vi "zherk - Hermitian Matrix Rank-k Update (CDB).vi"(4 "beta":dbl=1.0, 6 "alpha":dbl=1.0, 7 "operation A":T1 items=["Direct", "Conjugated & Transposed", "Transposed"], 8 "matrix C type":T2=3 items=["Lower Triangular"=2, "Upper Triangular"=3], 9 "C":T3, 11 "A":T3) -> (0 "error":i32, 3 "zherk":T3)   [LabVIEW 2017, in "NI_AALBLAS.lvlib"]
doc: "Calculates the rank-k update of the upper or lower triangular component of a Hermitian matrix."
uses:
  <vilib>/Analysis/NI_AALBLAS.lvlib
  <vilib>/Analysis/Matrix/Datatypes/ComplexMatrix.ctl
  <vilib>/Analysis/BLAS.llb/LV_UpLo.ctl
  <vilib>/Analysis/BLAS.llb/LV_Transpose.ctl
  <vilib>/Analysis/BLAS.llb/Fucntion.ctl
  <vilib>/Analysis/BLAS.llb/Order.ctl
  <vilib>/Analysis/BLAS.llb/BLAS3 Utility(CDB).vi
  <vilib>/Analysis/Matrix/NI_Matrix.lvlib
panel:
  # "zherk=alpha*A*conjg(A')+beta*C / zherk=alpha*conjg(A')*A+beta*C"
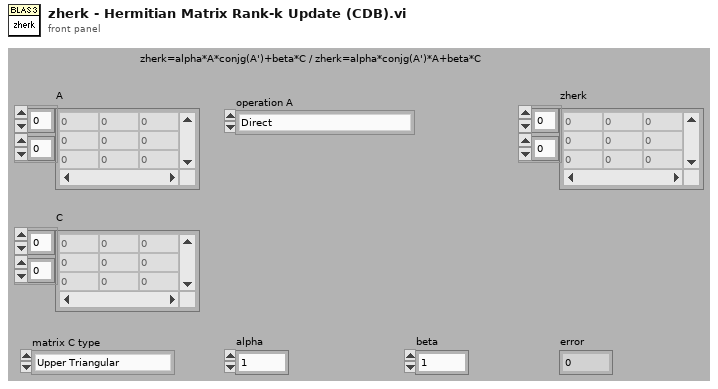
[diagram p1: front panel]
types:
  T1 = typedef "NI_AALBLAS.lvlib/LV_Transpose.ctl" = i32
  T2 = typedef "NI_AALBLAS.lvlib/LV_UpLo.ctl" = i32
  T3 = typedef "NI_Matrix.lvlib/ComplexMatrix.ctl" = cdb[][]
  T4 = typedef "NI_AALBLAS.lvlib/Order.ctl" = i32
  T5 = typedef "NI_AALBLAS.lvlib/Fucntion.ctl" = u16
  T6 = typedef "NI_AALBLAS.lvlib/Operation_Transpose.ctl" = i32
  T7 = typedef "NI_AALBLAS.lvlib/UpLo.ctl" = i32
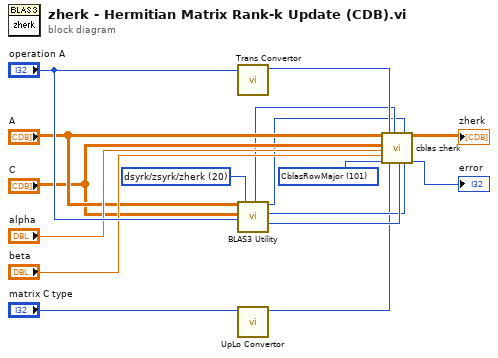
[diagram p0: block diagram]
diagram:
  w4 = T4 101 items=["CblasRowMajor"=101, "CblasColMajor"=102] ("order")
  w7 = T5 20 items=["ddot/zdotu/zdotc", "daxpy/zaxpy", "dnrm2/dznrm2", "dasum/dzasum", "dcopy/zcopy", "dswap/zswap", "drotm", "drot/zdrot", "idamax/izamax", "idamin/izamin", "dgemv/zgemv", "dsymv/zhemv", "dtrmv/ztrmv", "dsyr/zher", "dsyr2/zher2", "dger/zgeru/zgerc", "dtrsv/ztrsv", "dgemm/zgemm", "dsymm/zsymm/zhemm", "dtrmm/ztrmm", "dsyrk/zsyrk/zherk", "dsyr2k/zsyr2k/zher2k", "dtrsm/ztrsm"] ("function")
  n1 = call <vilib>:"Trans Convertor.vi"("operation"="operation A") -> ("trans"=w12:T6)  [unwired: 10 out]
  n2 = call-poly <vilib>:"BLAS3 Utility.vi"("A"="A", "C"="C", "operation A"="operation A", "function"=w7) -> ("lda"=w6:i32, "n"=w3:i32, "ldc"=w5:i32, "k"=w2:i32)  [unwired: 2 in, 10 out]
  n3 = call <vilib>:"UpLo Convertor.vi"("triangle matrix type"="matrix C type") -> ("uplo"=w1:T7)  [unwired: 10 out]
  n4 = call <vilib>:"cblas zherk.vi"("A"="A", "C"="C", "alpha"="alpha", "beta"="beta", "order"=w4, "transA"=w12, "uplo"=w1, "lda"=w6, "n"=w3, "ldc"=w5, "k"=w2) -> ("zherk"=→"zherk":T3, "error"=→"error":i32)  [unwired: 7 out]
